vi "PathPlanner_Path_FromJSON.vi"(11 "JSON String":string) -> (0 "Error":bool, 3 "PathPlannerPath":T1={"BezierPoints"=[], "PreviewStartingRotation"={"VALUE"=0.0, "COS"=1.0, "SIN"=0.0}, "Reversed"=FALSE, "RotationTargets"=[], "ConstraintZones"=[], "EventMarkers"=[], "GlobalConstraints"={"MaxVelocityMps;"=0.0, "MaxAccelerationMpsSq;"=0.0, "MaxAngularVelRadPsEc;"=0.0, "MaxAngularAccRadPSecSq"=0.0, "Exists"=FALSE}, "GoalEndState"={"Velocity"=0.0, "Rotation"={"VALUE"=0.0, "COS"=1.0, "SIN"=0.0}}, "AllPoints"=[]} {"AllPoints"."HolonomicRotation"."SIN" format="%13.4f"; "AllPoints"."HolonomicRotation"."COS" format="%13.4f"; "AllPoints"."HolonomicRotation"."VALUE" format="%13.4f"; "AllPoints"."Position"."Y" format="%14.3f"; "AllPoints"."Position"."X" format="%14.3f"; "GoalEndState"."Rotation"."SIN" format="%13.4f"; "GoalEndState"."Rotation"."COS" format="%13.4f"; "GoalEndState"."Rotation"."VALUE" format="%13.4f"; "EventMarkers"."lastRobotPos"."Y" format="%14.3f"; "EventMarkers"."lastRobotPos"."X" format="%14.3f"; "EventMarkers"."markerPos"."Y" format="%14.3f"; "EventMarkers"."markerPos"."X" format="%14.3f"; "RotationTargets"."target"."SIN" format="%13.4f"; "RotationTargets"."target"."COS" format="%13.4f"; "RotationTargets"."target"."VALUE" format="%13.4f"; "PreviewStartingRotation"."SIN" format="%13.4f"; "PreviewStartingRotation"."COS" format="%13.4f"; "PreviewStartingRotation"."VALUE" format="%13.4f"; "BezierPoints"."Y" format="%14.3f"; "BezierPoints"."X" format="%14.3f"})   [LabVIEW 2019, in "PathPlanner24.lvlib"]
uses:
  PathPlanner24.lvlib
  TypeDef/PathPlannerPath.ctl
  <vilib>/Rock Robotics/WPI/ThirdParty/JAS_Junk/TrajLib/TypeDef/TRANSLATION2D.ctl
  <vilib>/Rock Robotics/WPI/ThirdParty/JAS_Junk/TrajLib/TypeDef/ROTATION2D.ctl
  TypeDef/PathPlannerRotationTarget.ctl
  TypeDef/PathPlannerConstraintsZone.ctl
  TypeDef/PathPlannerPathConstraints.ctl
  TypeDef/PathPlannerEventMarker.ctl
  TypeDef/PathPlannerCommand.ctl
  TypeDef/PathPlannerGoalEndState.ctl
  TypeDef/PathPlannerPathPoint.ctl
  <vilib>/Rock Robotics/WPI/ThirdParty/JAS_Junk/TrajLib/Conv_Deg_Radians.vi
  <vilib>/Rock Robotics/WPI/ThirdParty/JAS_Junk/TrajLib/Rotation2d_CreateAngle.vi
  PathPlanner_GoalEndState_New.vi
  PathPlanner_PathConstraints_New.vi
  PathPlanner_EventMarker_New.vi
  PathPlanner_ConstraintsZone_New.vi
  PathPlanner_RotationTarget_New.vi
  <vilib>/Rock Robotics/WPI/ThirdParty/JAS_Junk/TrajLib/Trajectory_Library.lvlib
panel:
  in  "previewStartingState":cluster{"rotation":dbl}
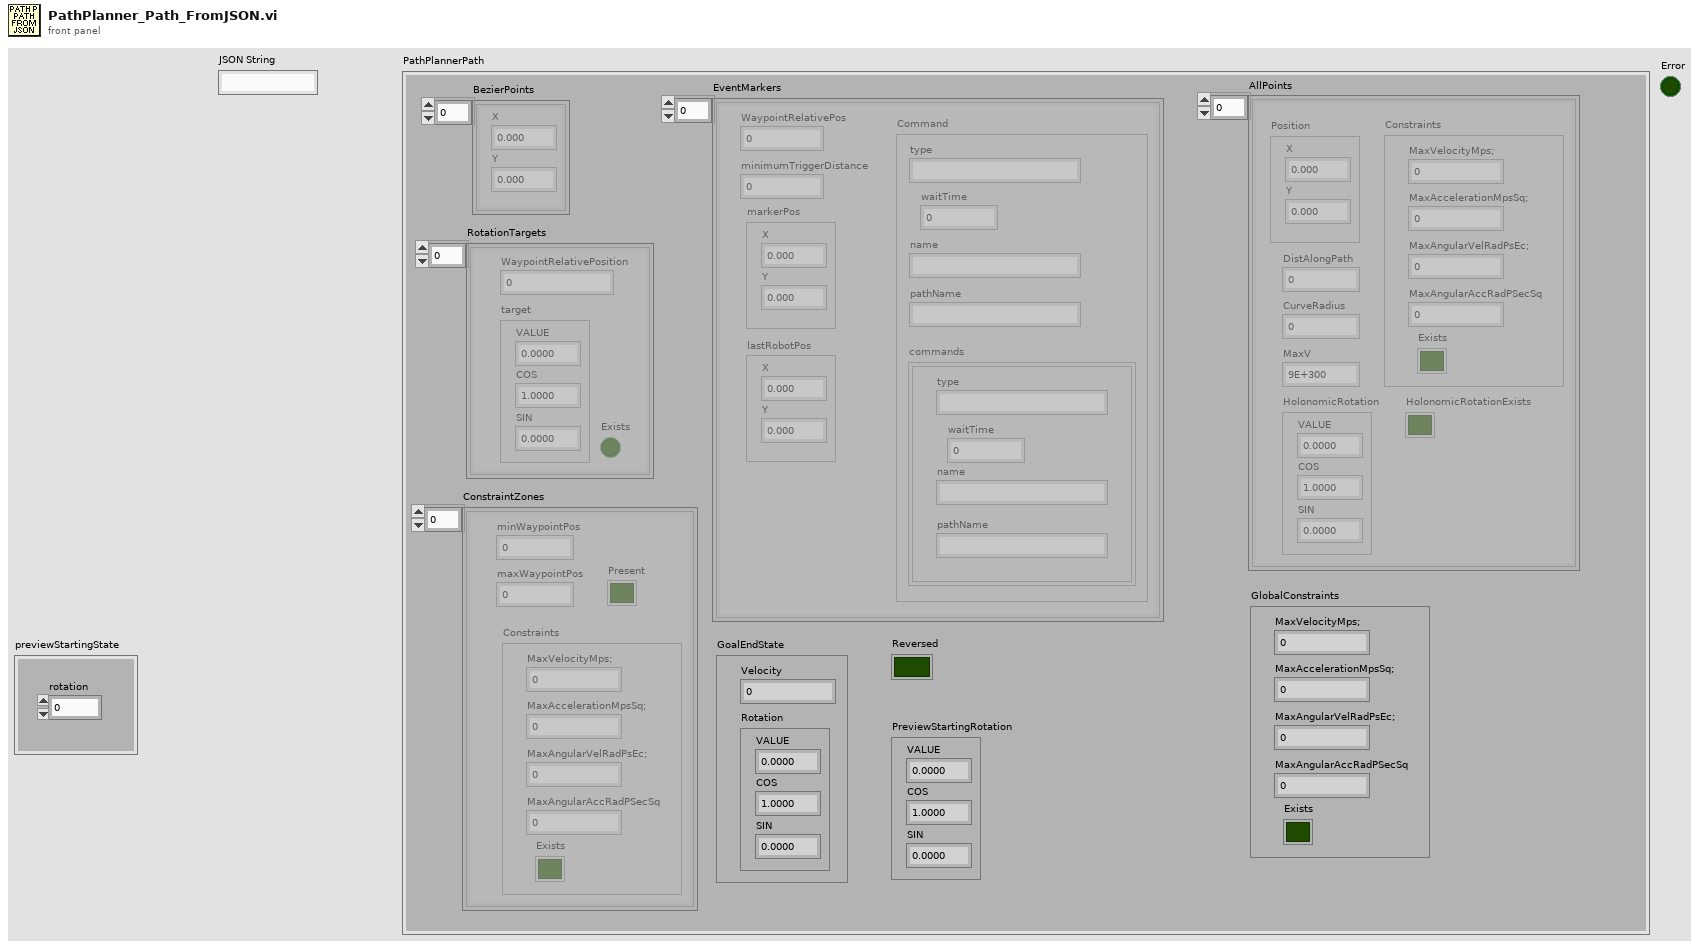
[diagram p1: front panel]
types:
  T1 = typedef "PathPlanner24.lvlib/PathPlannerPath.ctl" = cluster{"BezierPoints":T2[], "PreviewStartingRotation":T3, "Reversed":bool, "RotationTargets":T4[], "ConstraintZones":T5[], "EventMarkers":T7[], "GlobalConstraints":T6, "GoalEndState":T9, "AllPoints":T10[]}
  T2 = typedef "Trajectory_Library.lvlib/TRANSLATION2D.ctl" = cluster{"X":dbl, "Y":dbl}
  T3 = typedef "Trajectory_Library.lvlib/ROTATION2D.ctl" = cluster{"VALUE":dbl, "COS":dbl, "SIN":dbl}
  T4 = typedef "PathPlanner24.lvlib/PathPlannerRotationTarget.ctl" = cluster{"target":T3, "WaypointRelativePosition":dbl, "Exists":bool}
  T5 = typedef "PathPlanner24.lvlib/PathPlannerConstraintsZone.ctl" = cluster{"minWaypointPos":dbl, "maxWaypointPos":dbl, "Constraints":T6, "Present":bool}
  T6 = typedef "PathPlanner24.lvlib/PathPlannerPathConstraints.ctl" = cluster{"MaxVelocityMps;":dbl, "MaxAccelerationMpsSq;":dbl, "MaxAngularVelRadPsEc;":dbl, "MaxAngularAccRadPSecSq":dbl, "Exists":bool}
  T7 = typedef "PathPlanner24.lvlib/PathPlannerEventMarker.ctl" = cluster{"WaypointRelativePos":dbl, "minimumTriggerDistance":dbl, "markerPos":T2, "lastRobotPos":T2, "Command":T8}
  T8 = typedef "PathPlanner24.lvlib/PathPlannerCommand.ctl" = cluster{"waitTime":dbl, "name":string, "type":string, "pathName":string, "commands":cluster{"type":string, "waitTime":dbl, "name":string, "pathName":string}[]}
  T9 = typedef "PathPlanner24.lvlib/PathPlannerGoalEndState.ctl" = cluster{"Velocity":dbl, "Rotation":T3}
  T10 = typedef "PathPlanner24.lvlib/PathPlannerPathPoint.ctl" = cluster{"Position":T2, "HolonomicRotation":T3, "DistAlongPath":dbl, "CurveRadius":dbl, "MaxV":dbl, "Constraints":T6, "HolonomicRotationExists":bool}
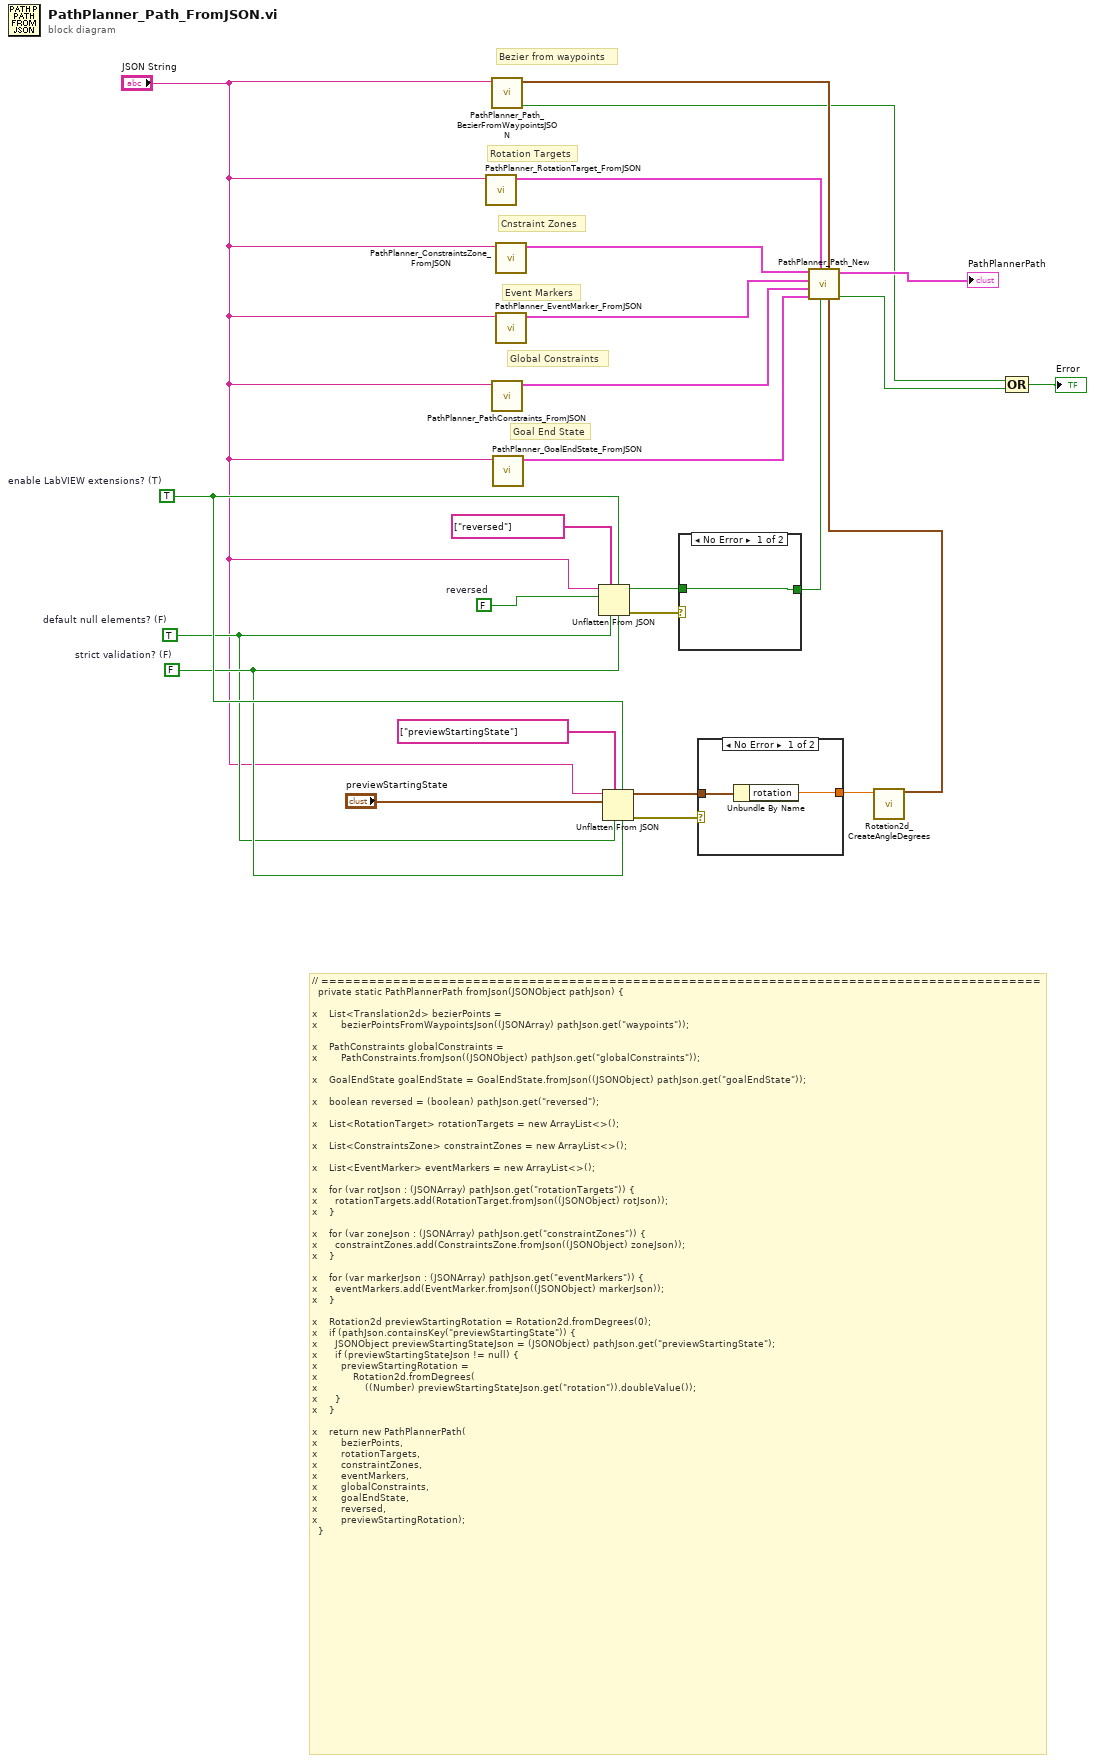
[diagram p0: block diagram]
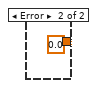
[diagram p2: hidden frame]
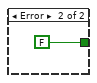
[diagram p3: hidden frame]
diagram:
  w13 = FALSE  # strict validation? (F)
  w12 = TRUE  # default null elements? (F)
  w14 = TRUE  # enable LabVIEW extensions? (T)
  w18 = FALSE  # reversed
  # "Bezier from waypoints"
  # "Goal End State"
  # "Global Constraints"
  # "Event Markers"
  # "Cnstraint Zones"
  # "Rotation Targets"
  # "// ==========================================================================================\n  private static PathPlannerPath fromJson(JSONObject pathJson) {\n\nx    List<Translation2d> bezierPoints =\nx        bezierPointsFromWaypointsJson((JSONArray) pathJson.get(\"waypoints\"));\n\nx    PathConstraints globalConstraints =\nx        PathConstraints.fromJson((JSONObject) pathJson.get(\"globalConstraints\"));\n\nx    GoalEndState goalEndState = GoalEndState.fromJson((JSONObject) pathJson.get(\"goalEndState\"));\n\nx    boolean reversed = (boolean) pathJson.get(\"reversed\");\n\nx    List<RotationTarget> rotationTargets = new ArrayList<>();\n\nx    List<ConstraintsZone> constraintZones = new ArrayList<>();\n\nx    List<EventMarker> eventMarkers = new ArrayList<>();\n\nx    for (var rotJson : (JSONArray) pathJson.get(\"rotationTargets\")) {\nx      rotationTargets.add(RotationTarget.fromJson((JSONObject) rotJson));\nx    }\n\nx    for (var zoneJson : (JSONArray) pathJson.get(\"constraintZones\")) {\nx      constraintZones.add(ConstraintsZone.fromJson((JSONObject) zoneJson));\nx    }\n\nx    for (var markerJson : (JSONArray) pathJson.get(\"eventMarkers\")) {\nx      eventMarkers.add(EventMarker.fromJson((JSONObject) markerJson));\nx    }\n\nx    Rotation2d previewStartingRotation = Rotation2d.fromDegrees(0);\nx    if (pathJson.containsKey(\"previewStartingState\")) {\nx      JSONObject previewStartingStateJson = (JSONObject) pathJson.get(\"previewStartingState\");\nx      if (previewStartingStateJson != null) {\nx        previewStartingRotation =\nx            Rotation2d.fromDegrees(\nx                ((Number) previewStartingStateJson.get(\"rotation\")).doubleValue());\nx      }\nx    }\n\nx    return new PathPlannerPath(\nx        bezierPoints,\nx        rotationTargets,\nx        constraintZones,\nx        eventMarkers,\nx        globalConstraints,\nx        goalEndState,\nx        reversed,\nx        previewStartingRotation);\n  }"
  n1 = call "PathPlanner_RotationTarget_FromJSON.vi"("JSON String"="JSON String") -> ("RotationTargets"=w25:T4[])  [unwired: 9 in, 1 out]
  n2 = call "PathPlanner_Path_BezierFromWaypointsJSON.vi"("JSON string"="JSON String") -> ("Error"=w1:bool, "Bezier"=w2:T2[])  [unwired: 8 in, 1 out]
  n3 = call "PathPlanner_PathConstraints_FromJSON.vi"("JSON String"="JSON String") -> ("PathPlannerConstraints"=w22:T6)  [unwired: 9 in, 1 out]
  n4 = call "PathPlanner_GoalEndState_FromJSON.vi"("JSON String"="JSON String") -> ("GoalEndState"=w21:T9)  [unwired: 9 in, 1 out]
  n5 = call "PathPlanner_ConstraintsZone_FromJSON.vi"("JSON String"="JSON String") -> ("ConstraintZones"=w24:T5[])  [unwired: 9 in, 1 out]
  n6 = call "PathPlanner_EventMarker_FromJSON.vi"("JSON String"="JSON String") -> ("EventMarkers"=w23:T7[])  [unwired: 9 in, 1 out]
  n7 = Unflatten From JSON(path=string[] ["reversed"] ("path 3"), enable LabVIEW extensions? (T)=w14, JSON string="JSON String", type and defaults=w18, default null elements? (F)=w12, strict validation? (F)=w13) -> (value=w8:bool, error out=w10:errorcluster)  [unwired: 1 in]
  n8 = Unflatten From JSON(path=string[] ["previewStartingState"] ("path 3"), enable LabVIEW extensions? (T)=w14, JSON string="JSON String", type and defaults="previewStartingState", default null elements? (F)=w12, strict validation? (F)=w13) -> (value=w6:cluster{"rotation":dbl}, error out=w7:errorcluster)  [unwired: 1 in]
  n9 = case shown="No Error" w10 {
    tunnel: [w26 FALSE] -> w9
    tunnel: w8 -> [w26 _]
    frame No Error {
    }
    frame Error {
    }
  }
  n10 = case shown="No Error" w7 {
    tunnel: [w28 0.0] -> w5
    tunnel: w6 -> [w29 _]
    frame No Error {
      n11 = Unbundle By Name(w29) -> ("rotation"=w28:dbl)
    }
    frame Error {
    }
  }
  n12 = call <vilib>:"Rotation2d_CreateAngleDegrees.vi"("Angle_Degrees"=w5) -> ("ROTATION"=w4:T3)  [unwired: 10 in]
  n13 = call "PathPlanner_Path_New.vi"("PreviewStartingRotation"=w4, "BezierPoints"=w2, "Reversed"=w9, "HolonomicRotations"=w25, "GoalEndState"=w21, "GlobalConstraints"=w22, "EventMarkers"=w23, "ConstraintZones"=w24) -> ("Error"=w17:bool, "PathPlannerPath"=→"PathPlannerPath":T1)  [unwired: 2 in]
  n14 = Compound Arithmetic op=OR(w1, w17) -> (→"Error":bool)
